vi "New.vi"(8 "error in (no error)":errorcluster, 11 "DoublyNode in":refnum<class "DoublyNode.lvclass">) -> (0 "error out":errorcluster, 2 "data value reference":refnum<data-value>, 3 "DoublyNode out":refnum<class "DoublyNode.lvclass">)   [LabVIEW 2021, in "DoublyNode.lvclass"]
uses:
  DoublyNode.lvclass
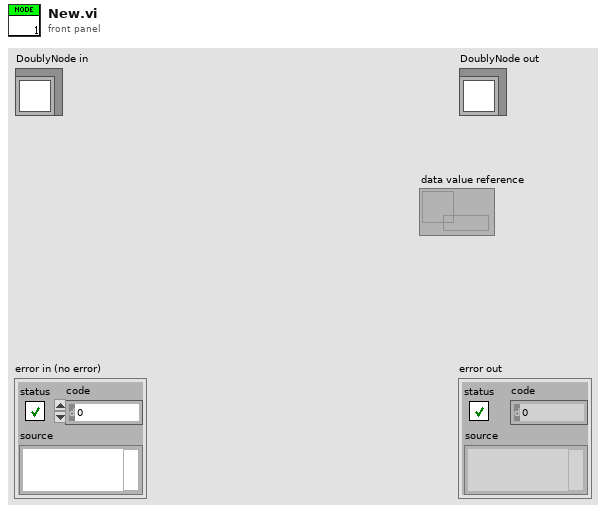
[diagram p1: front panel]
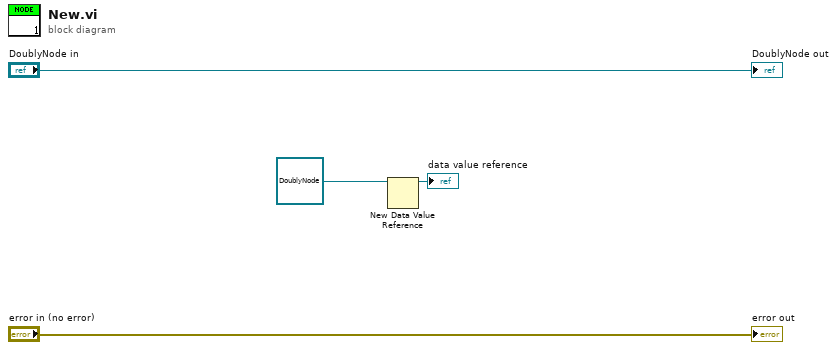
[diagram p0: block diagram]
diagram:
  n1 = New Data Value Reference(data value=refnum<class "DoublyNode.lvclass"> refnum ("DoublyNode.lvclass")) -> (data value reference=→"data value reference":refnum<data-value>)  [unwired: 1 in, 1 out]
  "error out" <- "error in (no error)"
  "DoublyNode out" <- "DoublyNode in"
